vi "Histogram_cumulative.vi"() -> ()   [LabVIEW 2010]
uses:
  <vilib>/Analysis/NI_AALPro.lvlib
panel:
  out "Array 2":i32[](array[numeric])
  out "Array":i32[](array[numeric])
  in  "# bins":i32
  out "XY Graph":cluster{"Axis":dbl[], i32[]}(graph)
  out "Histogram Graph":T1(graph)
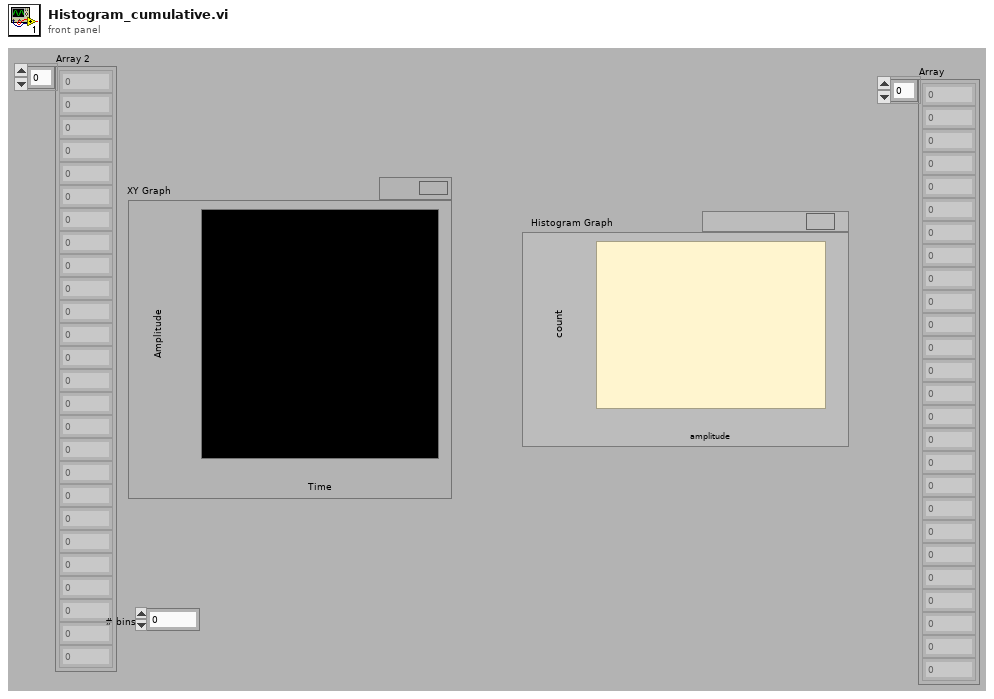
[diagram p1: front panel]
types:
  T1 = cluster{"X Values":dbl[], "Histogram: h(x)":i32[]}
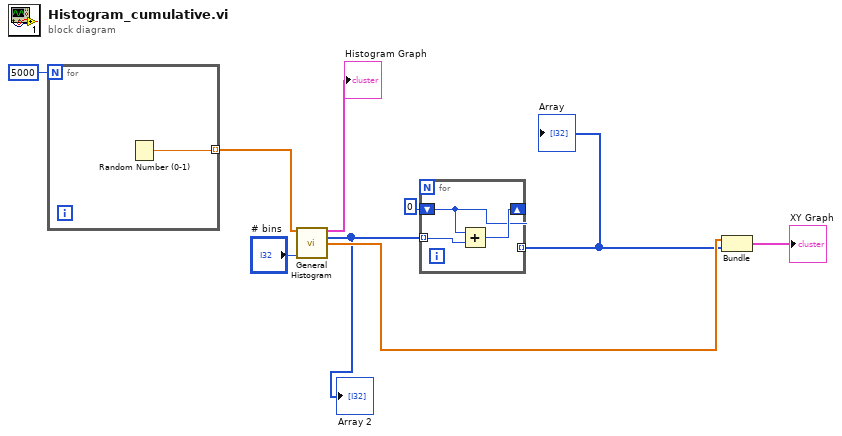
[diagram p0: block diagram]
diagram:
  n1 = for {
    N: 5000 -> [_]
    tunnel: [w10] -> w9 mode=indexing
    n2 = Random Number (0-1)() -> (number: 0 to 1=w10:dbl)
  }
  n3 = call <vilib>:"General Histogram.vi"("X"=w9, "# bins"="# bins") -> ("Histogram Graph"=→"Histogram Graph":T1, "Histogram"=w1:i32[], "Axis"=w4:dbl[])  [unwired: 9 in, 2 out]
  "Array 2" <- w1
  n4 = for {
    tunnel: w1 -> [w13] mode=indexing
    shift-right: [w12] -> _
    shift-left: 0 -> [w11]
    tunnel: [w11] -> w3 mode=indexing
    n5 = Add(x=w11, y=w13) -> (x+y=w12:i32)
  }
  "Array" <- w3
  n6 = Bundle("Axis"=w4, w3) -> (→"XY Graph":cluster{"Axis":dbl[], i32[]})  [unwired: 1 in]
